vi "写入Beverage.lvclass.vi"(8 "error in (no error)":errorcluster caption="错误输入（无错误）", 10 "Beverage.lvclass":refnum<class "Beverage.lvclass">, 11 "Mocha输入":refnum<class "Mocha.lvclass">) -> (0 "error out":errorcluster caption="错误输出", 3 "Mocha输出":refnum<class "Mocha.lvclass">)   [LabVIEW 2016, in "Mocha.lvclass"]
uses:
  Mocha.lvclass
  Beverage.lvclass
  Mocha.lvclass/Mocha.ctl
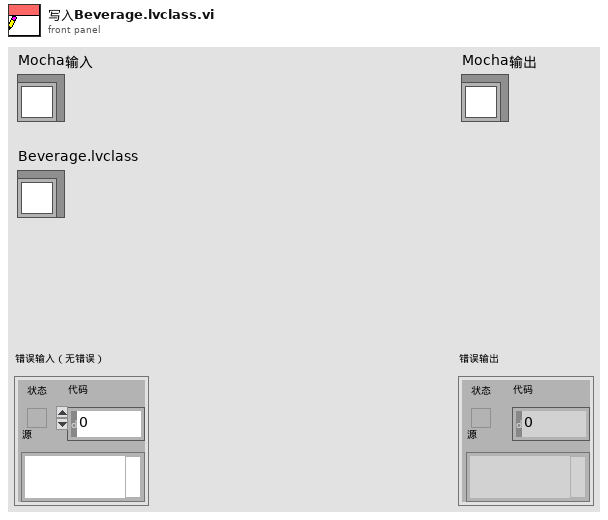
[diagram p1: front panel]
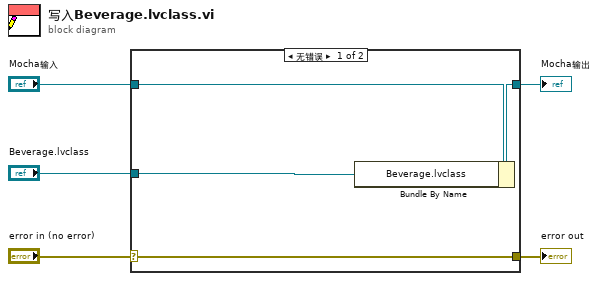
[diagram p0: block diagram]
diagram:
  n1 = case shown="无错误" "error in (no error)" {
    selector: "error in (no error)" -> [w9 w10]
    tunnel: [w9 w10] -> w4
    tunnel: [w7 w11] -> w2
    tunnel: "Mocha输入" -> [w8 w11]
    tunnel: "Beverage.lvclass" -> [w6 _]
    frame No Error {
      n2 = Bundle By Name(cluster=w8, "Beverage.lvclass"=w6) -> (w7:refnum<class "Mocha.lvclass">)
    }
    frame Error {
    }
  }
  "error out" <- w4
  "Mocha输出" <- w2
